vi "ECAT FPGA OD FoE.vi"(8 "error in":errorcluster, 10 "Product Code":u32, 11 "Input bitfile path":path) -> (0 "error out":errorcluster, 1 "OD object structure":T1[](array[typedef]) {"od_index" format="%.0x"; "lptr_name" format="%.0x"; "lptr_data" format="%.0x"; "lptr_entry" format="%.0x"; "DataInfo"."u8Array" format="%.0x"}, 2 "IOVs from bitfile":T2(array[cluster]) {"address" format="%.0x"}, 3 "Output Byte array":u8[](array[numeric]) max=0)   [LabVIEW 2019, in "SEECD System Explorer.lvlib"]
uses:
  SEECD System Explorer.lvlib
  <vilib>/LabVIEW Targets/FPGA/ECat/subVIs/FPGAParsingVIs/niECATODInfoStructure.ctl
  <vilib>/Utility/sysdir.llb/Get System Directory.vi
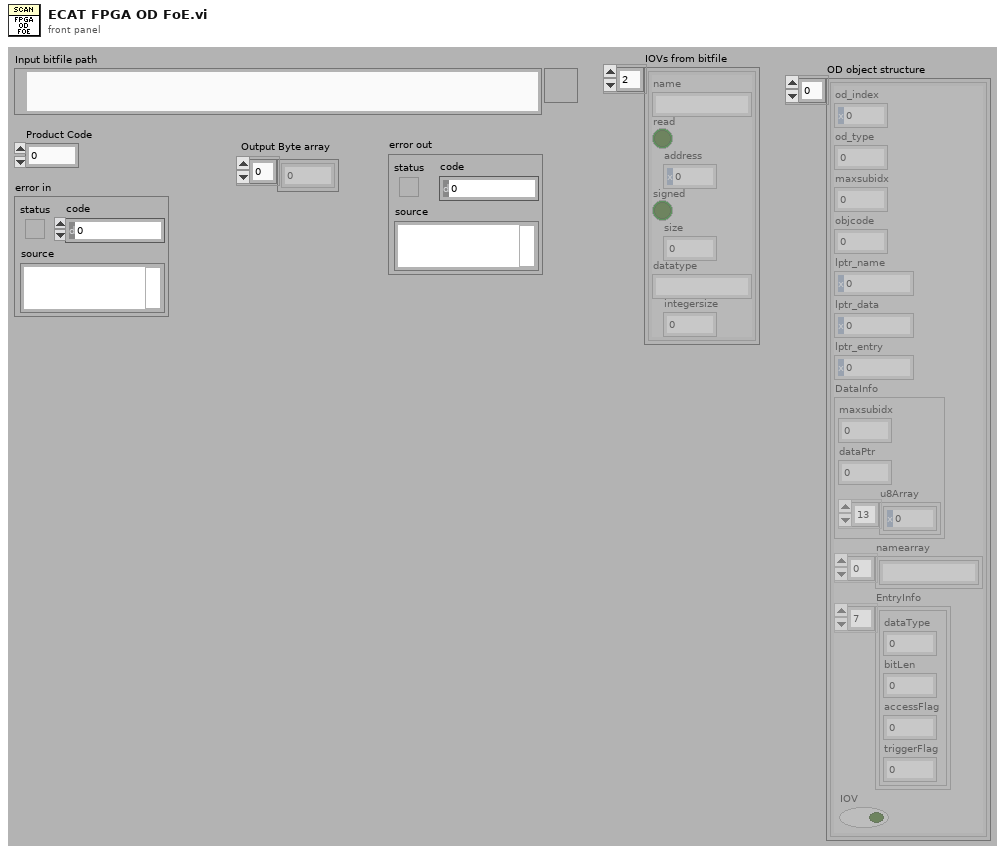
[diagram p1: front panel]
types:
  T1 = typedef "niECATODInfoStructure.ctl" = cluster{"od_index":u32, "od_type":u16, "maxsubidx":u8, "objcode":u8, "lptr_name":u32, "lptr_data":u32, "lptr_entry":u32, "DataInfo":cluster{"maxsubidx":u32, "dataPtr":u32, "u8Array":u8[]}, "namearray":string[], "EntryInfo":cluster{"dataType":u16, "bitLen":u16, "accessFlag":u16, "triggerFlag":u16}[], "IOV":bool}
  T2 = cluster{"name":string, "read":bool, "address":u32, "signed":bool, "size":u32, "datatype":string, "integersize":i32}[]
  T3 = typedef "niECATFXPInfoStruct.ctl" = cluster{"name":string, "ODIndex":u32, "integersize":i32, "wordsize":u32, "Signed":bool}
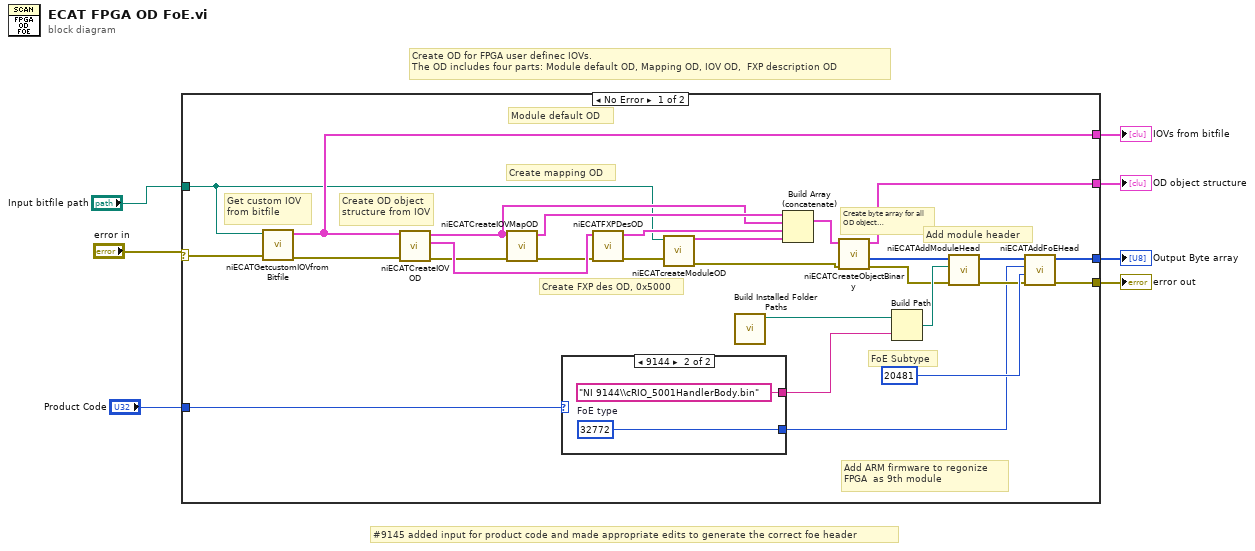
[diagram p0: block diagram]
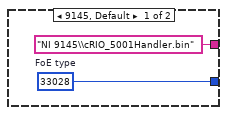
[diagram p2: hidden frame]
diagram:
  # "#9145 added input for product code and made appropriate edits to generate the correct foe header"
  # "Create OD for FPGA user definec IOVs. \nThe OD includes four parts: Module default OD, Mapping OD, IOV OD,  FXP description OD"
  n1 = case shown="No Error" "error in" {
    selector: "error in" -> [w23 w39]
    tunnel: "Input bitfile path" -> [w13 _]
    tunnel: [w24 _] -> w6
    tunnel: [w19 _] -> w4
    tunnel: [w18 _] -> w3
    tunnel: [w14 w39] -> w2
    tunnel: "Product Code" -> [w11 _]
    frame No Error {
      # "Add ARM firmware to regonize\nFPGA  as 9th module"
      # "Module default OD"
      # "Create FXP des OD, 0x5000"
      # "Create mapping OD"
      # "Create byte array for all OD object \nstructure from IOV"
      # "Create OD object \nstructure from IOV"
      # "FoE Subtype"
      # "Add module header"
      # "Get custom IOV\nfrom bitfile"
      n2 = call <vilib>:"niECATGetcustomIOVfromBitfile.vi"("error in"=w23, "Input bitfile path"=w13) -> ("error out"=w22:errorcluster, "User defined IOVs"=w19:T2)  [unwired: 8 in]
      n3 = call <vilib>:"niECATCreateIOVOD.vi"("error in"=w22, "Input IOV info Array"=w19) -> ("error out"=w21:errorcluster, "FXP Info"=w27:T3[], "ObjectODArray"=w28:T1[])  [unwired: 7 in]
      n4 = call <vilib>:"niECATCreateIOVMapOD.vi"("error in"=w21, "IOV OD structure"=w28) -> ("error out"=w20:errorcluster, "IOV map OD structure"=w29:T1[])  [unwired: 8 in]
      n5 = case shown="9144" w11 {
        tunnel: [w36 w38] -> w9
        tunnel: ["NI 9145\\cRIO_5001Handler.bin" ("name or relative path") "NI 9144\\cRIO_5001HandlerBody.bin" ("name or relative path")] -> w10
        frame 9145, Default {
          w36 = u16 33028  # FoE type
        }
        frame 9144 {
          w38 = u16 32772  # FoE type
        }
      }
      n6 = call <vilib>:"niECATFXPDesOD.vi"("error in"=w20, "FXP Info Array"=w27) -> ("error out"=w17:errorcluster, "FXPODs"=w26:T1[])  [unwired: 8 in]
      n7 = call <vilib>:"niECATcreateModuleOD.vi"("error in"=w17, "Input bitfile path"=w13) -> ("error out"=w16:errorcluster, "Module OD array"=w12:T1[])  [unwired: 8 in]
      n8 = call "Build Installed Folder Paths.vi"() -> ("Data Folder Path"=w8:path)  [unwired: 10 in, 1 out]
      n9 = Build Array (concatenate)(w29, w28, w26, w12) -> (w30:T1[])
      n10 = call <vilib>:"niECATCreateObjectBinary.vi"("error in"=w16, "Object structure array"=w30) -> ("error out"=w15:errorcluster, "Object byte array"=w31:u8[], "Object structure array"=w18:T1[])  [unwired: 6 in, 1 out]
      n11 = Build Path(base path=w8, name or relative path=w10) -> (appended path=w32:path)
      n12 = call <vilib>:"niECATAddModuleHead.vi"("error in"=w15, "ARM firmware path"=w32, "Input byte Array"=w31) -> ("error out"=w25:errorcluster, "Output module array"=w34:u8[])  [unwired: 7 in]
      n13 = call <vilib>:"niECATAddFoEHead.vi"("error in"=w25, "Subtype"=u16 20481, "Type"=w9, "Input FoE body Byte array"=w34) -> ("error out"=w14:errorcluster, "Output Byte array with FoE head"=w24:u8[])  [unwired: 6 in]
    }
    frame Error {
    }
  }
  "error out" <- w2
  "Output Byte array" <- w6
  "IOVs from bitfile" <- w4
  "OD object structure" <- w3
